vi "Elevator Control Loop - Motion Profile.vi"() -> ()   [LabVIEW 2014, in "Elevator System.lvlib"]
uses:
  Elevator System.lvlib
  <vilib>/Rock Robotics/WPI/MotorControl/WPI_MotorControlDeviceRef.ctl
  <vilib>/Rock Robotics/WPI/MotorControl/WPI_MotorControlType.ctl
  <vilib>/Rock Robotics/SystemInterfaces/Typedef/FPGA_TypedefDigitalModule.ctl
  <vilib>/Rock Robotics/SystemInterfaces/DIO/FPGA_DIOPWMChannel.ctl
  <vilib>/Rock Robotics/WPI/PWM/WPI_PWMDeadband.ctl
  <vilib>/Rock Robotics/WPI/CAN/Jaguar/SubVIs/WPI_CANJaguar_ControlMode.ctl
  <vilib>/Rock Robotics/WPI/CAN/TalonSRX/WPI_CANTalonSRX_APIControlMode.ctl
  <vilib>/Rock Robotics/WPI/PWM/WPI_PWMTransform_ConPane.ctl
  Typedef/FGVAction.ctl
  <vilib>/Platform/TimedLoop/XDataNode/timing_clust.ctl
  <vilib>/Platform/TimedLoop/XDataNode/nitl_modes.ctl
  <vilib>/Platform/TimedLoop/XDataNode/wakeup.ctl
  Public/StupidGlobal.vi
  <vilib>/addons/control/pid/pid.llb/PID (DBL).vi
  SimulatorVIs/Simulation Input Global.vi
  <vilib>/platform/TimedLoop/XDataNode/XDataNode.xnode
  <vilib>/addons/control/pid/NI_PID_pid.lvlib
  <vilib>/Platform/TimedLoop/XDataNode/XDNodeRunTimeDep.lvlib
panel:
  in  "Up speed":dbl=0.8 format="%#_13g"
  in  "Down Speed":dbl=-0.65 format="%#_13g"
  in  "upper limit":dbl=1.0
  in  "lower limit":dbl=-1.0
  in  "G Constant":dbl=0.05
  in  "FeedForward Kv":dbl=0.5
  in  "Max Velocity":dbl=70.0
  in  "Max Acceleration":dbl=8.0
  out "Plant Input":dbl(graph)=0.1293337112592495
  in  "output range":cluster{"output high":dbl, "output low":dbl}={"output high"=1.0, "output low"=-1.0} {"output low" format="%.2f"; "output high" format="%.2f"}
  in  "PID gains":T1={"proportional gain (Kc)"=1.0, "integral time (Ti, min)"=1.0, "derivative time (Td, min)"=0.0} {"derivative time (Td, min)" format="%.3f"; "integral time (Ti, min)" format="%.3f"; "proportional gain (Kc)" format="%.3f"}
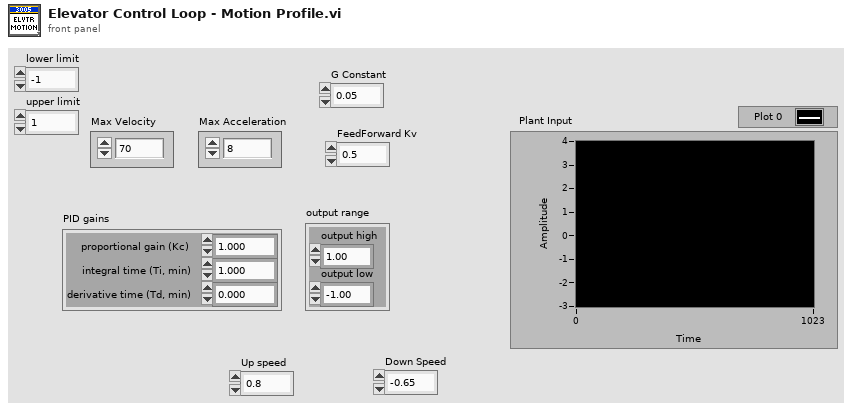
[diagram p1: front panel]
types:
  T1 = cluster{"proportional gain (Kc)":dbl, "integral time (Ti, min)":dbl, "derivative time (Td, min)":dbl}
  T2 = typedef "Elevator System.lvlib/FGVAction.ctl" = enum16{"get", "set"}
  T3 = typedef "WPI_MotorControlDeviceRef.ctl" = cluster{"DeviceStatus":errorcluster, "Type":T4, "PWM":cluster{"Controller":T5, "PWM Channel":T6, "DeadBand":T7}, "CAN":cluster{"Device Number":u8, "Control Mode":T8, "Semaphore":T9, "Max Vout":dbl, "TalonSRX Control Mode":T10}, "Invert":bool, "TransformRef":T11, "InvTransformRef":T11}
  T4 = typedef "WPI_MotorControlType.ctl" = enum16{"PWM", "CAN", "CANTalonSRX"}
  T5 = typedef "FPGA_TypedefDigitalModule.ctl" = enum16{"Controller 1"}
  T6 = typedef "FPGA_DIOPWMChannel.ctl" = enum8{"PWM 0", "PWM 1", "PWM 2", "PWM 3", "PWM 4", "PWM 5", "PWM 6", "PWM 7", "PWM 8", "PWM 9", "PWM MXP 0", "PWM MXP 1", "PWM MXP 2", "PWM MXP 3", "PWM MXP 4", "PWM MXP 5", "PWM MXP 6", "PWM MXP 7", "PWM MXP 8", "PWM MXP 9", "Invalid"}
  T7 = typedef "WPI_PWMDeadband.ctl" = cluster{"Name":string, "maxPositivePwm":i32, "minPositivePwm":i32, "centerPwm":i32, "maxNegativePwm":i32, "minNegativePwm":i32, "angularRange":u16}
  T8 = typedef "WPI_CANJaguar_ControlMode.ctl" = enum8{"Percent VBus", "Current", "Speed", "Position", "Voltage"}
  T9 = typedef "Semaphore RefNum" = refnum<k1>
  T10 = typedef "WPI_CANTalonSRX_APIControlMode.ctl" = enum8{"Percent VBus", "Speed", "Position", "Slave", "Unchanged / Invalid"}
  T11 = typedef "WPI_PWMTransform_ConPane.ctl" = refnum<vi>
  T12 = cluster{"Setpoint":dbl, "notifier out":refnum<notifier>, "Output":dbl, "DriveMotor":T3, "Position":dbl, "SP Profile":cluster{"Position":dbl[], "Velocity":dbl[], "Time":dbl[]}, "Counter":i64}
  T13 = typedef "WPI_PotentiometerDevRef.ctl" = cluster{"DevStatus":errorcluster, "Controller":T14, "Analog Channel":T15, "Invert Output":bool}
  T14 = typedef "FPGA_TypedefAnalogModule.ctl" = enum16{"Controller 1"}
  T15 = typedef "FPGA_AIChannel.ctl" = enum8{"AI 0", "AI 1", "AI 2", "AI 3", "AI MXP 0", "AI MXP 1", "AI MXP 2", "AI MXP 3", "Invalid"}
  T16 = typedef "XDNodeRunTimeDep.lvlib/timing_clust.ctl" = cluster{"Expected End [f-1]":u64, "Actual End [f-1]":u64, "Finished Late? [f-1]":bool, "Expected End [i-1]":u64, "Actual End [i-1]":u64, "Finished Late? [i-1]":bool, "Expected Start [i]":u64, "Actual Start [i]":u64, "Expected Start [f]":u64, "Actual Start [f]":u64, "Source Name":string, "Structure Name":string, "Period":i64, "Deadline":i64, "Offset":i64, "Start":i64, "Priority":i32, "Timeout":i32, "Mode":T17, "Wakeup Reason":T18, "Error":errorcluster, "Source Type":string, "Secondary Source Type":string, "Global End Time":u64, "Global Start Time":u64, "Frame Duration":u64, "Iteration Duration":u64, "Assigned CPU":i32, "I/O Scan Engine Mode":u32}
  T17 = typedef "XDNodeRunTimeDep.lvlib/nitl_modes.ctl" = enum32{"No Change", "Process missed periods, maintain original phase", "Discard missed periods, maintain original phase", "Process missed periods, ignore original phase", "Discard missed periods, ignore original phase"}
  T18 = typedef "XDNodeRunTimeDep.lvlib/wakeup.ctl" = enum32{"Normal", "Aborted", "Asynchronous wakeup", "Timing source error", "Timed loop error", "Timeout"}
  T19 = cluster{"Position":dbl[], "Velocity":dbl[], "Time":dbl[]}
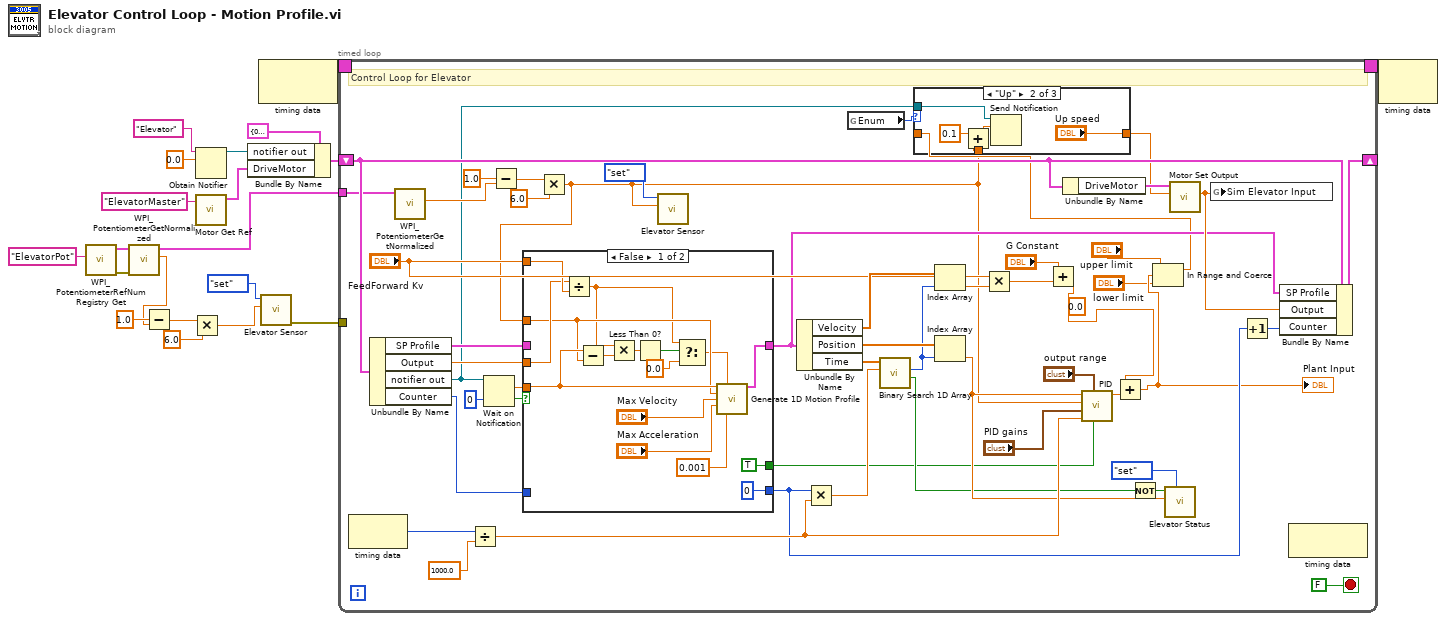
[diagram p0: block diagram]
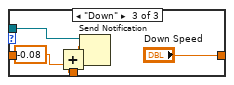
[diagram p3: hidden frame]
diagram:
  n1 = call <vilib>:"WPI_PotentiometerRefNum Registry Get.vi"("refnum name"="ElevatorPot") -> ("error out"=w5:errorcluster, "PotDevRef"=w4:T13)  [unwired: 9 in]
  n2 = call <vilib>:"WPI_PotentiometerGetNormalized.vi"("error in"=w5, "PotDevRef"=w4) -> ("Normalized Value"=w2:dbl, "PotDevRef"=w3:T13)  [unwired: 7 in, 1 out]
  n3 = Subtract(x=1.0, y=w2) -> (x-y=w9:dbl)
  n4 = Multiply(x=w9, y=6.0) -> (x*y=w7:dbl)
  n5 = Obtain Notifier(name (unnamed)="Elevator", notification data type=0.0 ("Setpoint")) -> (notifier out=w18:refnum<notifier>)  [unwired: 2 in, 2 out]
  n6 = call "Motor Get Ref.vi"("refnum name"="ElevatorMaster") -> ("MotorControlDevRef"=w15:T3)  [unwired: 10 in]
  n7 = Bundle By Name(cluster=T12 {"Setpoint"=0.0, "notifier out"=refnum, "Output"=0.0, "DriveMotor"={"DeviceStatus"={"status"=FALSE, "code"=0, "source"=""}, "Type"=enum."PWM", "PWM"={"Controller"=enum."Controller 1", "PWM Channel"=enum."Invalid", "DeadBand"={"Name"="", "maxPositivePwm"=0, "minPositivePwm"=0, "centerPwm"=0, "maxNegativePwm"=0, "minNegativePwm"=0, "angularRange"=0}}, "CAN"={"Device Number"=0, "Control Mode"=enum."Percent VBus", "Semaphore"=refnum, "Max Vout"=12.0, "TalonSRX Control Mode"=enum."Percent VBus"}, "Invert"=FALSE, "TransformRef"=refnum, "InvTransformRef"=refnum}, "Position"=0.0, "SP Profile"={"Position"=[], "Velocity"=[], "Time"=[]}, "Counter"=0}, "notifier out"=w18, "DriveMotor"=w15) -> (w19:T12)
  n8 = node-c288() -> (w13:T16)  [unwired: 1 in]
  n9 = call "Elevator Sensor.vi"("Value"=w7, "Action"=FGVAction."set") -> ("error out"=w1:errorcluster)  [unwired: 8 in, 1 out]
  n10 = timed-loop {
    shift-right: [w68] -> _
    shift-left: w19 -> [w60]
    timing: w13 -> [_]
    timing-out: [_] -> w12
    tunnel: w3 -> [w30]
    tunnel: w1 -> [_]
    stop <- FALSE stop-if-true
    (unwired) 0.0 ("t")
    # "Control Loop for Elevator"
    n11 = node-c288() -> (w53:i64)  [unwired: 1 in]
    n12 = Unbundle By Name(w60) -> ("SP Profile"=w61:T19, "Output"=w63:dbl, "notifier out"=w22:refnum<notifier>, "Counter"=w55:i64)
    n13 = call <vilib>:"WPI_PotentiometerGetNormalized.vi"("PotDevRef"=w30) -> ("Normalized Value"=w33:dbl)  [unwired: 8 in, 2 out]
    n14 = Divide(x=w53, y=1000.0) -> (x/y=w48:dbl)
    n15 = Wait on Notification(notifier=w22, timeout in ms (-1)=0) -> (notification=w64:dbl, timed out?=w65:bool)  [unwired: 2 in, 2 out]
    n16 = Subtract(x=1.0, y=w33) -> (x-y=w35:dbl)
    n17 = Multiply(x=w35, y=6.0) -> (x*y=w21:dbl)
    n18 = case shown="False" w65 {
      tunnel: w64 -> [w92 _]
      tunnel: "FeedForward Kv" -> [w97 _]
      tunnel: w63 -> [w96 _]
      tunnel: w61 -> [_ w101]
      tunnel: [w95 w101] -> w41
      tunnel: w55 -> [_ w100]
      tunnel: [i64 0 ("Counter") w100] -> w42
      tunnel: w21 -> [w91 _]
      tunnel: [TRUE _] -> w31
      frame False {
        # "New SP Given"
        n19 = Divide(x=w96, y=w97) -> (x/y=w87:dbl)
        n20 = Subtract(x=w92, y=w91) -> (x-y=w90:dbl)
        n21 = Multiply(x=w87, y=w90) -> (x*y=w89:dbl)
        n22 = Less Than 0?(x=w89) -> (x < 0?=w88:bool)
        n23 = Select(t=w87, s=w88, f=0.0) -> (s? t:f=w85:dbl)
        n24 = call "Generate 1D Motion Profile.vi"("Target Position"=w92, "Initial Velocity (0)"=w85, "Initial Position (0)"=w91, "Max Velocity"="Max Velocity", "Max Acceleration"="Max Acceleration", "resolution m (.001)"=0.001) -> ("Time Plot"=w95:T19)  [unwired: 7 in, 2 out]
      }
      frame True {
      }
    }
    n25 = call "Elevator Sensor.vi"("Value"=w21, "Action"=FGVAction."set") -> ()  [unwired: 8 in, 2 out]
    n26 = Unbundle By Name(w41) -> ("Velocity"=w51:dbl[], "Position"=w50:dbl[], "Time"=w56:dbl[])
    n27 = Multiply(x=w42, y=w48) -> (x*y=w52:dbl)
    n28 = global read "StupidGlobal.vi" "Enum"() -> (w24:enum16{"Down", "Up", "Auto"})
    n29 = call "Binary Search 1D Array.vi"("element"=w52, "1D array sorted"=w56) -> ("Path Complete?"=w38:bool, "index"=w49:i32)  [unwired: 7 in, 1 out]
    n30 = Index Array(array=w51, index=w49) -> (element=w46:dbl)
    n31 = Index Array(array=w50, index=w49) -> (element=w39:dbl)
    n32 = Multiply(x="FeedForward Kv", y=w46) -> (x*y=w44:dbl)
    n33 = Add(x="G Constant", y=w44) -> (x+y=w26:dbl)
    n34 = Unbundle By Name(w60) -> ("DriveMotor"=w66:T3)
    n35 = call-poly <vilib>:"PID.vi"("reinitialize? (F)"=w31, "output range"="output range", "dt (s)"=w48, "PID gains"="PID gains", "process variable"=w21, "setpoint"=w39) -> ("output"=w47:dbl)  [unwired: 4 in, 1 out]
    n36 = Add(x=w26, y=w47) -> (x+y=w29:dbl)
    "Plant Input" <- w29
    n37 = Not(x=w38) -> (.not. x?=w37:bool)
    n38 = In Range and Coerce(upper limit="upper limit", x=w29, lower limit="lower limit") -> (coerced(x)=w25:dbl)  [unwired: 1 out]
    n39 = case shown="\"Up\"" w24 {
      tunnel: w25 -> [w70 _ _]
      tunnel: [w70 "Up speed" "Down Speed"] -> w23
      tunnel: w22 -> [_ w74 w78]
      tunnel: w21 -> [_ w73 w79]
      frame "Auto", Default {
      }
      frame "Up" {
        n40 = Add(x=0.1, y=w73) -> (x+y=w72:dbl)
        n41 = Send Notification(notification=w72, notifier=w74) -> ()  [unwired: 1 in, 2 out]
      }
      frame "Down" {
        n42 = Add(x=w79, y=-0.08 ("x")) -> (x+y=w77:dbl)
        n43 = Send Notification(notification=w77, notifier=w78) -> ()  [unwired: 1 in, 2 out]
      }
    }
    n44 = call "Elevator Status.vi"("Action"=FGVAction."set", "Input"=w39, "Moving? (F)"=w37) -> ()  [unwired: 6 in, 3 out]
    n45 = call "Motor Set Output.vi"("output"=w23, "DriveMotor"=w66) -> ("Motor Output"=w62:dbl)  [unwired: 9 in]
    n46 = global write "Simulation Input Global.vi" "Sim Elevator Input"(w62) -> ()
    n47 = Increment(x=w42) -> (x+1=w43:i64)
    n48 = Bundle By Name(cluster=w60, "SP Profile"=w41, "Output"=w62, "Counter"=w43) -> (w68:T12)
    n49 = node-c288() -> ()  [unwired: 1 in, 1 out]
  }
  n50 = node-c288(w12) -> ()  [unwired: 1 out]
